vi "SerialPort_ECS02.vi"(2 "error in (no error)":errorcluster, 3 "COM Port":refnum<visa-resource-name>) -> (0 "error out":errorcluster)   [LabVIEW 2014]
uses:
  <vilib>/Instr/_visa.llb/VISA Open Access Mode.ctl
  <vilib>/Instr/_visa.llb/VISA Configure Serial Port (Instr).vi
  g_Stop.vi
  g_ECS02_Command.vi
panel:
  in  "Timeout (ms)":i32=120
  out "Write":string
  out "read buffer":string
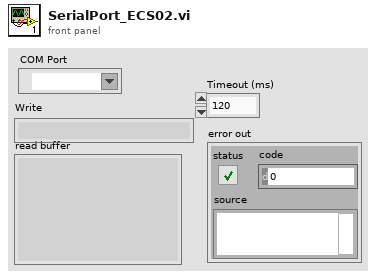
[diagram p1: front panel]
types:
  T1 = typedef "VISA Open Access Mode.ctl" = u32
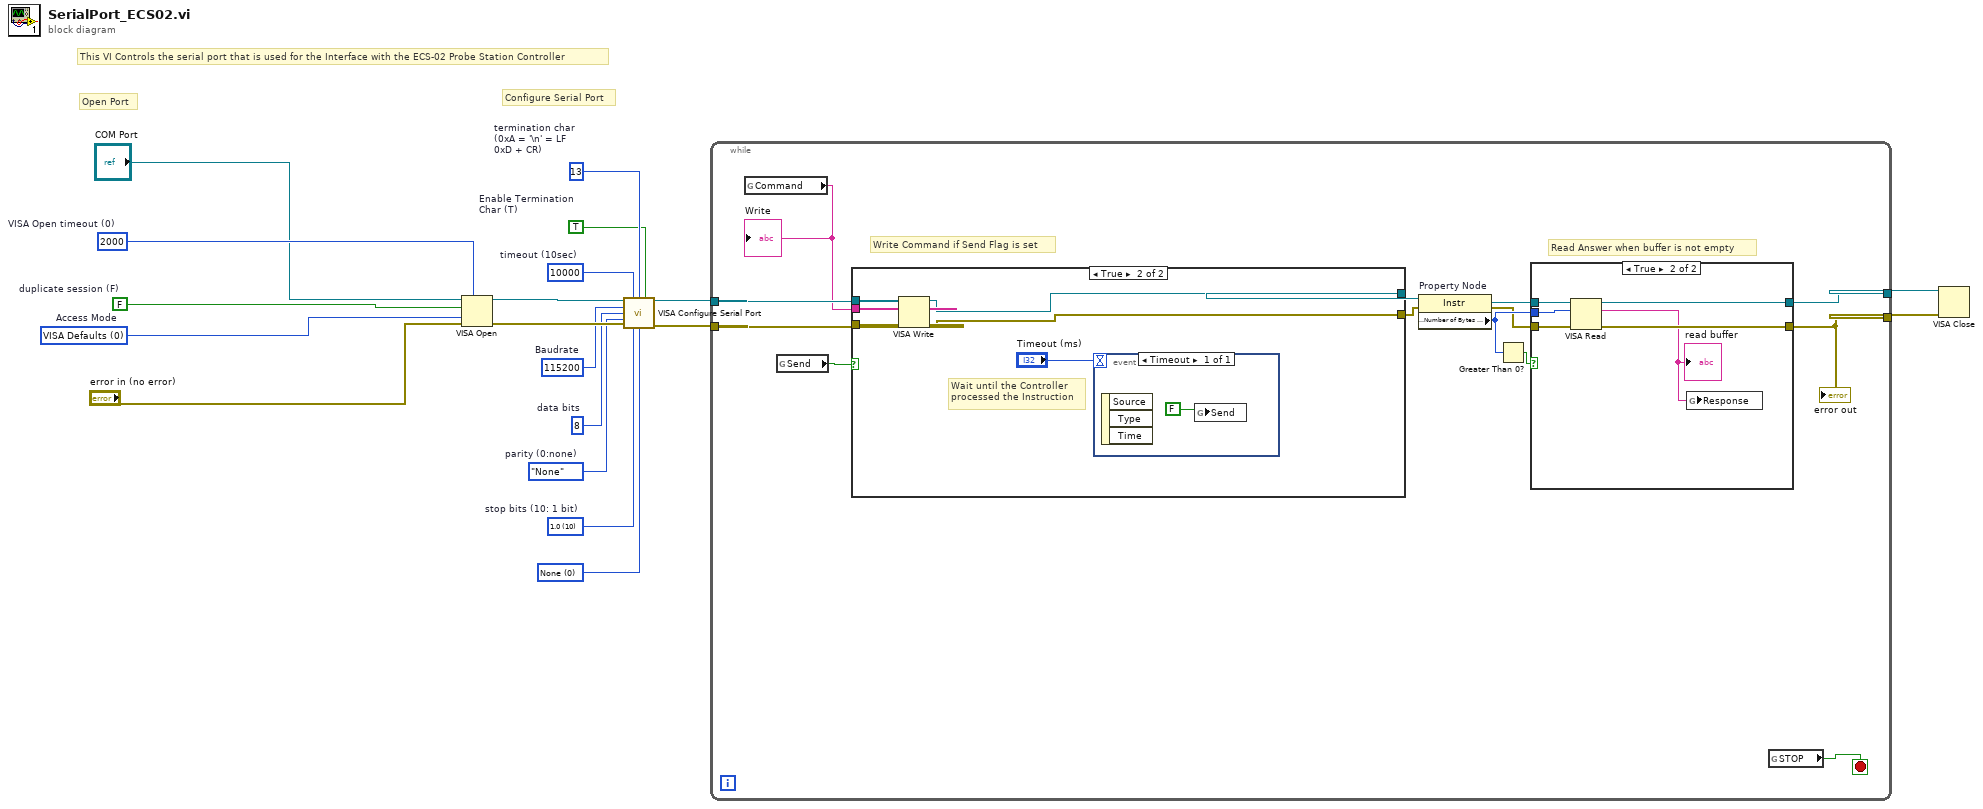
[diagram p0: block diagram]
diagram:
  w5 = u32 10000  # timeout (10sec)
  w6 = T1 0 items=["VISA Defaults"=0, "Exclusive Lock"=1, "Load Configured Settings"=4]  # Access Mode
  w7 = FALSE  # duplicate session (F)
  w10 = TRUE  # Enable Termination Char (T)
  w11 = u8 13  # termination char (0xA = '\n' = LF 0xD + CR)
  w12 = u16 0 items=["None", "XON/XOFF", "RTS/CTS", "XON/XOFF & RTS/CTS", "DTR/DSR", "XON/XOFF & DTR/DSR"] ("flow control (0:none)")
  w13 = u16 10 items=["1.0"=10, "1.5"=15, "2.0"=20]  # stop bits (10: 1 bit)
  w14 = enum16{"None", "Odd", "Even", "Mark", "Space"}."None"  # parity (0:none)
  w15 = u32 115200  # Baudrate
  w16 = u16 8  # data bits
  w18 = u32 2000  # VISA Open timeout (0)
  # "Configure Serial Port"
  # "This VI Controls the serial port that is used for the Interface with the ECS-02 Probe Station Controller"
  # "Open Port"
  n1 = VISA Open(timeout (0)=w18, duplicate session (F)=w7, access mode=w6, error in (no error)="error in (no error)", VISA resource name="COM Port") -> (VISA resource name=w19:refnum<visa-resource-name>, error out=w17:errorcluster)
  n2 = call-poly "VISA Configure Serial Port"("VISA resource name"=w19, "timeout (10sec)"=w5, "termination char\n(0xA = '\\n' = LF)"=w11, "Enable Termination\nChar (T)"=w10, "baud rate (9600)"=w15, "data bits (8)"=w16, "parity (0:none)"=w14, "error in (no error)"=w17, "stop bits (10: 1 bit)"=w13, "flow control (0:none)"=w12) -> ("VISA resource name out"=w9:refnum<visa-resource-name>, "error out"=w8:errorcluster)  [unwired: 4 in]
  n3 = while {
    tunnel: w9 -> [w30]
    tunnel: w8 -> [w29]
    tunnel: [w31] -> w4
    tunnel: [w32] -> w3
    stop <- w26 stop-if-true
    # "Read Answer when buffer is not empty"
    # "Write Command if Send Flag is set"
    n4 = global read "g_ECS02_Command.vi" "Command"() -> (w25:string)
    "Write" <- w25
    n5 = global read "g_ECS02_Command.vi" "Send"() -> (w22:bool)
    n6 = case shown="True" w22 {
      tunnel: w30 -> [w41 w48]
      tunnel: w29 -> [w42 w46]
      tunnel: w25 -> [_ w47]
      tunnel: [w42 w44] -> w21
      tunnel: [w41 w45] -> w23
      frame False {
      }
      frame True {
        # "Wait until the Controller \nprocessed the Instruction"
        n7 = VISA Write(VISA resource name=w48, write buffer=w47, error in (no error)=w46) -> (VISA resource name out=w45:refnum<visa-resource-name>, error out=w44:errorcluster)  [unwired: 1 out]
        n8 = event shown="[0] Timeout" {
          selector: _ -> [_]
          dyn-events: _ -> [_]
          timeout: "Timeout (ms)" -> [_]
          event Timeout {
            n9 = event-data() -> ()  [unwired: 1 in, 3 out]
            n10 = global write "g_ECS02_Command.vi" "Send"(FALSE) -> ()
          }
        }
      }
    }
    n11 = property on="Property Node" class="Instr"(reference=w23, error in=w21) -> (reference out=w24:refnum<visa-resource-name>, error out=w20:errorcluster, "Serial Settings:Number of Bytes at Serial Port"=w27:u32)
    n12 = Greater Than 0?(x=w27) -> (x > 0?=w28:bool)
    n13 = case shown="True" w28 {
      tunnel: w24 -> [w34 w40]
      tunnel: w20 -> [w33 w39]
      tunnel: [w34 w38] -> w32
      tunnel: [w33 w37] -> w31
      tunnel: w27 -> [_ w36]
      frame False {
      }
      frame True {
        n14 = VISA Read(VISA resource name=w40, byte count=w36, error in (no error)=w39) -> (VISA resource name out=w38:refnum<visa-resource-name>, read buffer=w35:string, error out=w37:errorcluster)  [unwired: 1 out]
        "read buffer" <- w35
        n15 = global write "g_ECS02_Command.vi" "Response"(w35) -> ()
      }
    }
    "error out" <- w31
    n16 = global read "g_Stop.vi" "STOP"() -> (w26:bool)
  }
  n17 = VISA Close(VISA resource name=w3, error in (no error)=w4) -> ()  [unwired: 1 out]
